vi "Rotation Execute.vi"   [LabVIEW 2016]
uses:
  Rotation Control Type.ctl
  <vilib>/Rock Robotics/WPI/DriverStation/WPI_DriverStationRobotMode2.ctl
  Rotation Notifier.ctl
  Rotation Globals.vi
  Robot Global Data.vi
types:
  T1 = typedef "WPI_MotorControlDeviceRef.ctl" = cluster{"DeviceStatus":errorcluster, "Type":T2, "PWM":cluster{"PWM Channel":T3, "DeadBand":T4}, "CAN":cluster{"Device Number":u8, "SetOutput VI Ref":variant, "GetOutput VI Ref":variant, "Enable VI Ref":variant, "Disable VI Ref":variant, "Data":variant}, "Invert":bool}
  T2 = typedef "WPI_MotorControlType.ctl" = enum16{"PWM", "CAN"}
  T3 = typedef "FPGA_DIOPWMChannel.ctl" = enum8{"PWM 0", "PWM 1", "PWM 2", "PWM 3", "PWM 4", "PWM 5", "PWM 6", "PWM 7", "PWM 8", "PWM 9", "PWM MXP 0", "PWM MXP 1", "PWM MXP 2", "PWM MXP 3", "PWM MXP 4", "PWM MXP 5", "PWM MXP 6", "PWM MXP 7", "PWM MXP 8", "PWM MXP 9", "Invalid"}
  T4 = typedef "WPI_PWMDeadband.ctl" = cluster{"Name":string, "maxPositivePwm":i32, "minPositivePwm":i32, "centerPwm":i32, "maxNegativePwm":i32, "minNegativePwm":i32, "angularRange":u16}
  T5 = typedef "Rotation Control Type.ctl" = enum16{"No Op", "Up", "Down", "Control Up", "Control Down", "Gear Down", "Gear Up"}
  T6 = typedef "Rotation Notifier.ctl" = cluster{"Up":bool, "Down":bool, "Rotation Control List":T5, "Control Down":bool, "Manual":bool, "Parameter 1":dbl, "Parameter 2":dbl, "Rotation Notifier":refnum<notifier>, "Step":i32}
  T7 = typedef "WPI_DriverStationRobotMode2.ctl" = enum16{"Autonomous Disabled", "Autonomous Enabled", "Teleop Disabled", "Teleop Enabled", "Disconnected", "Finish", "Test Disabled", "Test Enabled", "Emergency Stopped"}
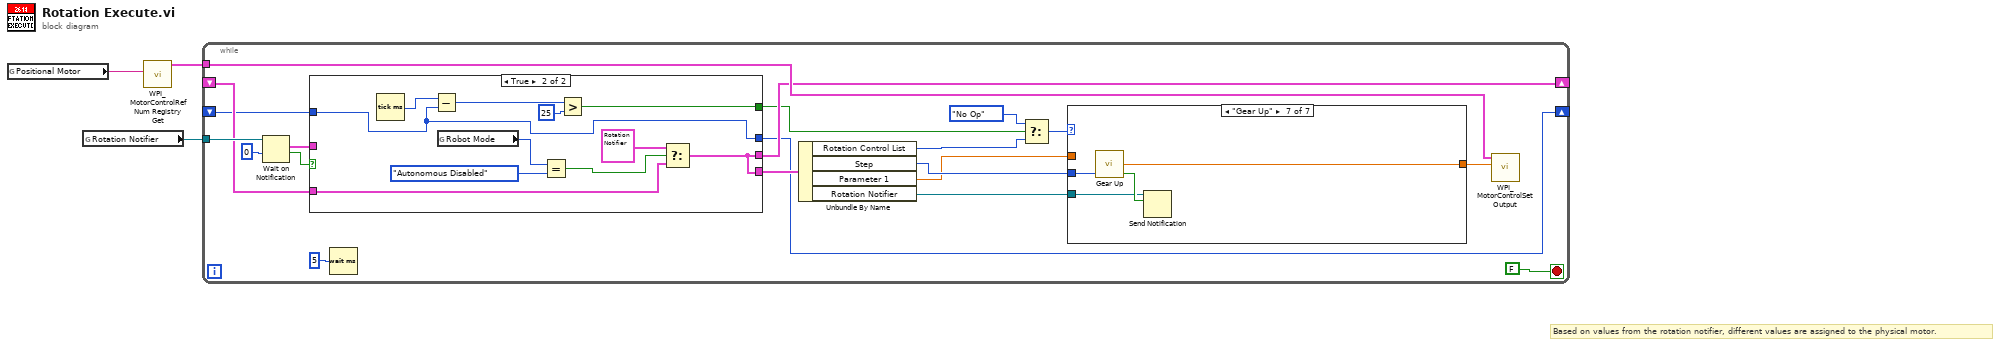
[diagram p0: block diagram]
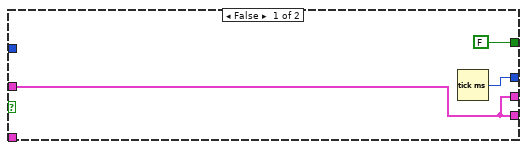
[diagram p2: hidden frame]
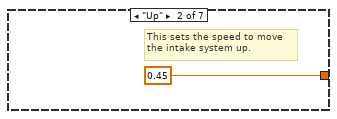
[diagram p4: hidden frame]
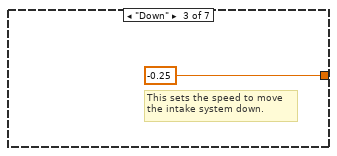
[diagram p5: hidden frame]
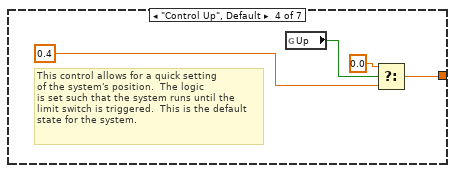
[diagram p6: hidden frame]
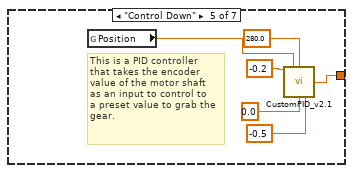
[diagram p7: hidden frame]
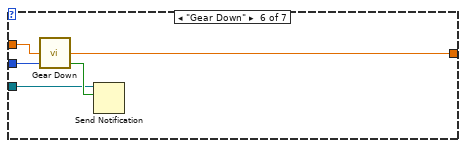
[diagram p8: hidden frame]
diagram:
  # "Based on values from the rotation notifier, different values are assigned to the physical motor."
  n1 = global read "Rotation Globals.vi" "Positional Motor"() -> (w1:string)
  n2 = global read "Rotation Globals.vi" "Rotation Notifier"() -> (w3:refnum<notifier>)
  n3 = call <vilib>:"WPI_MotorControlRefNum Registry Get.vi"("refnum name"=w1) -> ("MotorControlDevRef"=w2:T1)  [unwired: 9 in, 1 out]
  n4 = while {
    tunnel: w3 -> [w21]
    tunnel: w2 -> [w20]
    shift-right: [w14] -> _
    shift-left: _ -> [w13]
    shift-right: [w12] -> _
    shift-left: _ -> [w11]
    stop <- FALSE stop-if-true
    n5 = Wait on Notification(notifier=w21, timeout in ms (-1)=0) -> (notification=w16:T6, timed out?=w17:bool)  [unwired: 2 in, 2 out]
    n6 = case shown="True" w17 {
      tunnel: w16 -> [w26 _]
      tunnel: [w26 w28] -> w14
      tunnel: [w26 w28] -> w15
      tunnel: w13 -> [_ w29]
      tunnel: [w25 w36] -> w12
      tunnel: w11 -> [_ w36]
      tunnel: [FALSE w33] -> w7
      frame False {
        n7 = Tick Count (ms)() -> (millisecond timer value=w25:u32)
      }
      frame True {
        n8 = Tick Count (ms)() -> (millisecond timer value=w37:u32)
        n9 = Subtract(x=w37, y=w36) -> (x-y=w35:u32)
        n10 = global read "Robot Global Data.vi" "Robot Mode"() -> (w32:T7)
        n11 = Equal?(x=w32, y=WPI_DriverStationRobotMode2."Autonomous Disabled") -> (x = y?=w30:bool)
        n12 = Greater?(x=w35, y=u32 25) -> (0:w33:bool)
        n13 = Select(t=T6 {"Up"=FALSE, "Down"=FALSE, "Rotation Control List"=enum."No Op", "Control Down"=FALSE, "Manual"=FALSE, "Parameter 1"=0.0, "Parameter 2"=0.0, "Rotation Notifier"=refnum, "Step"=0} ("Rotation Notifier"), s=w30, f=w29) -> (s? t:f=w28:T6)
      }
    }
    n14 = Wait (ms)(milliseconds to wait=u32 5) -> ()  [unwired: 1 out]
    n15 = Unbundle By Name(w15) -> ("Rotation Control List"=w10:T5, "Step"=w6:i32, "Parameter 1"=w5:dbl, "Rotation Notifier"=w4:refnum<notifier>)
    n16 = Select(t=Rotation_Control_Type."No Op", s=w7, f=w10) -> (s? t:f=w9:T5)
    n17 = case shown="\"Gear Up\"" w9 {
      tunnel: [_ 0.45 ("Output") -0.25 ("Output") w40 w44 w52 w57] -> w19
      tunnel: w6 -> [_ _ _ _ _ w53 w58]
      tunnel: w5 -> [_ _ _ _ _ w54 _]
      tunnel: w4 -> [_ _ _ _ _ w50 w55]
      frame "No Op" {
      }
      frame "Up" {
        # "This sets the speed to move \nthe intake system up."
      }
      frame "Down" {
        # "This sets the speed to move \nthe intake system down."
      }
      frame "Control Up", Default {
        # "This control allows for a quick setting\nof the system's position.  The logic \nis set such that the system runs until the\nlimit switch is triggered.  This is the default\nstate for the system."
        n18 = global read "Rotation Globals.vi" "Up"() -> (w43:bool)
        n19 = Select(t=0.0, s=w43, f=0.4) -> (s? t:f=w40:dbl)
      }
      frame "Control Down" {
        # "This is a PID controller\nthat takes the encoder\nvalue of the motor shaft\nas an input to control to\na preset value to grab the\ngear."
        n20 = global read "Rotation Globals.vi" "Position"() -> (w48:dbl)
        n21 = call "CustomPID_v2.1.vi"("Kp"=-0.2, "Process Variable"=w48, "Goal"=280.0, "Max Ouput"=0.0, "Min Output"=-0.5) -> ("Command"=w44:dbl)  [unwired: 8 in, 2 out]
      }
      frame "Gear Down" {
        n22 = call "Gear Down.vi"("Step"=w53, "Acceptable Error"=w54) -> ("Completed"=w51:bool, "Output"=w52:dbl)  [unwired: 2 in]
        n23 = Send Notification(notification=w51, notifier=w50) -> ()  [unwired: 1 in, 2 out]
      }
      frame "Gear Up" {
        n24 = call "Gear Up.vi"("Step"=w58) -> ("Completed"=w56:bool, "Output"=w57:dbl)  [unwired: 3 in]
        n25 = Send Notification(notification=w56, notifier=w55) -> ()  [unwired: 1 in, 2 out]
      }
    }
    n26 = call <vilib>:"WPI_MotorControlSetOutput.vi"("Output"=w19, "MotorControlDevRef"=w20) -> ()  [unwired: 7 in, 3 out]
  }
